vi "Filter_GEA2_Log.vi"(0 "GEA2 Log":string, 5 "Data":variant, 9 "State":enum16{"Add to Log", "Clear", "Shutdown"}(ring), 11 "error in (no error)":errorcluster) -> (4 "GEA2 Log":string, 6 "Latest Message":string, 10 "Shutdown":bool, 15 "error out":errorcluster)   [LabVIEW 2021]
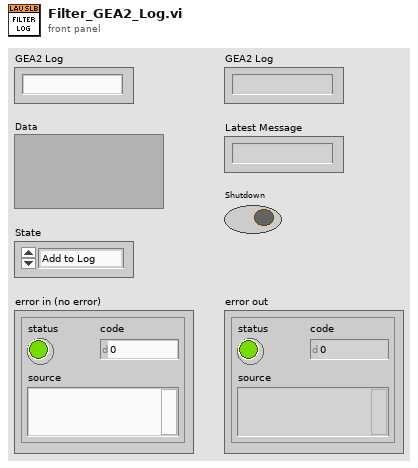
[diagram p1: front panel]
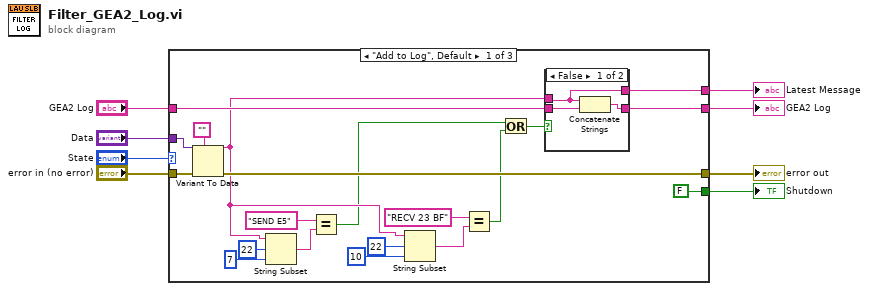
[diagram p0: block diagram]
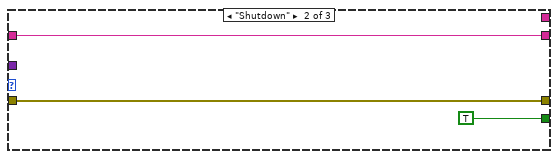
[diagram p3: hidden frame]
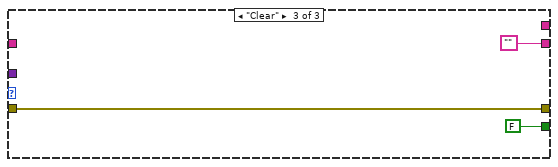
[diagram p4: hidden frame]
diagram:
  n1 = case shown="\"Add to Log\", Default" "State" {
    tunnel: "Data" -> [w25 _ _]
    tunnel: "GEA2 Log" -> [w28 w33 _]
    tunnel: [w27 w33 ""] -> w6
    tunnel: "error in (no error)" -> [w26 w34 w38]
    tunnel: [w23 w34 w38] -> w7
    tunnel: [FALSE TRUE FALSE] -> w5
    tunnel: [w17 _ _] -> w8
    frame "Add to Log", Default {
      n2 = Variant To Data(error in=w26, type="", Variant=w25) -> (data=w11:string, error out=w23:errorcluster)
      n3 = String Subset(string=w11, offset (0)=22, length (rest)=7 ("length (rest)")) -> (substring=w18:string)
      n4 = Equal?(x="SEND E5", y=w18) -> (x = y?=w9:bool)
      n5 = String Subset(string=w11, offset (0)=22, length (rest)=10 ("length (rest)")) -> (substring=w15:string)
      n6 = Equal?(x="RECV 23 BF", y=w15) -> (x = y?=w10:bool)
      n7 = Or(x=w9, y=w10) -> (x .or. y?=w16:bool)
      n8 = case shown="False" w16 {
        tunnel: w28 -> [w31 w32]
        tunnel: [w30 w32] -> w27
        tunnel: w11 -> [w29 _]
        tunnel: [w29 _] -> w17
        frame False {
          n9 = Concatenate Strings(w29, w31) -> (w30:string)
        }
        frame True {
        }
      }
    }
    frame "Shutdown" {
    }
    frame "Clear" {
    }
  }
  "Latest Message" <- w8
  "error out" <- w7
  "GEA2 Log" <- w6
  "Shutdown" <- w5
